vi "Metadata_Testing.vi"() -> ()   [LabVIEW 2016]
uses:
  <userlib>/LevyLab/Lockin-Multichannel/Typedefs/AO-cluster.ctl
  <userlib>/LevyLab/Lockin-Multichannel/Typedefs/AO_Amp-array.ctl
  <userlib>/LevyLab/Lockin-Multichannel/Typedefs/AO_DC-array.ctl
  <userlib>/LevyLab/Lockin-Multichannel/Typedefs/AO_f-array.ctl
  <userlib>/LevyLab/Lockin-Multichannel/Typedefs/AO_phi-array.ctl
  <userlib>/LevyLab/Lockin-Multichannel/Typedefs/Function-array.ctl
  <userlib>/LevyLab/Lockin-Multichannel/Typedefs/Function-enum.ctl
  levylab_expt_transport/src/SMOs/SweepControl/Typedefs/ScanParamters.ctl
  levylab_expt_transport/src/SMOs/SweepControl/Typedefs/Cluster - ScanParamters.ctl
  levylab_expt_transport/src/SMOs/SweepControl/Typedefs/PostAction.ctl
  levylab_expt_transport/src/SMOs/SweepControl/Typedefs/Enum - PostAction.ctl
  levylab_expt_transport/src/SMOs/SweepControl/Typedefs/ScanControl.ctl
  levylab_expt_transport/src/SMOs/SweepControl/Typedefs/Cluster - ScanControl.ctl
  levylab_expt_transport/src/SMOs/SweepControl/Typedefs/Enum - Priority.ctl
  levylab_expt_transport/src/SMOs/SweepControl/Typedefs/Enum - Action.ctl
  levylab_expt_transport/src/subVI/SweepMetadataV2.ctl
  levylab_expt_transport/src/SMOs/SweepControl/SweepControl.lvclass
panel:
  out "Sweep Metadata Cluster":T1 {"Channels: AO"."AO f (Hz)" min=0.001 max=10000.0; "Channels: AO"."AO DC (V)" format="%#_6p"; "Channels: AO"."AO amp (V)" format="%#_6p"}
  out "output cluster":T17 {"Sorted scan parameters"."?"."Rate" format="%.2f"; "Sorted scan parameters"."?"."Step" format="%#_6p"; "Sorted scan parameters"."?"."End" format="%#_6p"; "Sorted scan parameters"."?"."Start" format="%#_6p"}
  in  "<FROM SCAN CONTROL>":T18 {"Channels: AO"."AO f (Hz)" min=0.001 max=10000.0; "Channels: AO"."AO DC (V)" format="%#_6p"; "Channels: AO"."AO amp (V)" format="%#_6p"; "Scan parameters"."Rate" format="%.2f"; "Scan parameters"."Step" format="%#_6p"; "Scan parameters"."End" format="%#_6p"; "Scan parameters"."Start" format="%#_6p"}
  # "0"
  # "1"
  # "2"
  # "3"
  # "4"
  # "5"
  # "6"
  # "7"
  # "0"
  # "1"
  # "2"
  # "3"
  # "4"
  # "5"
  # "6"
  # "7"
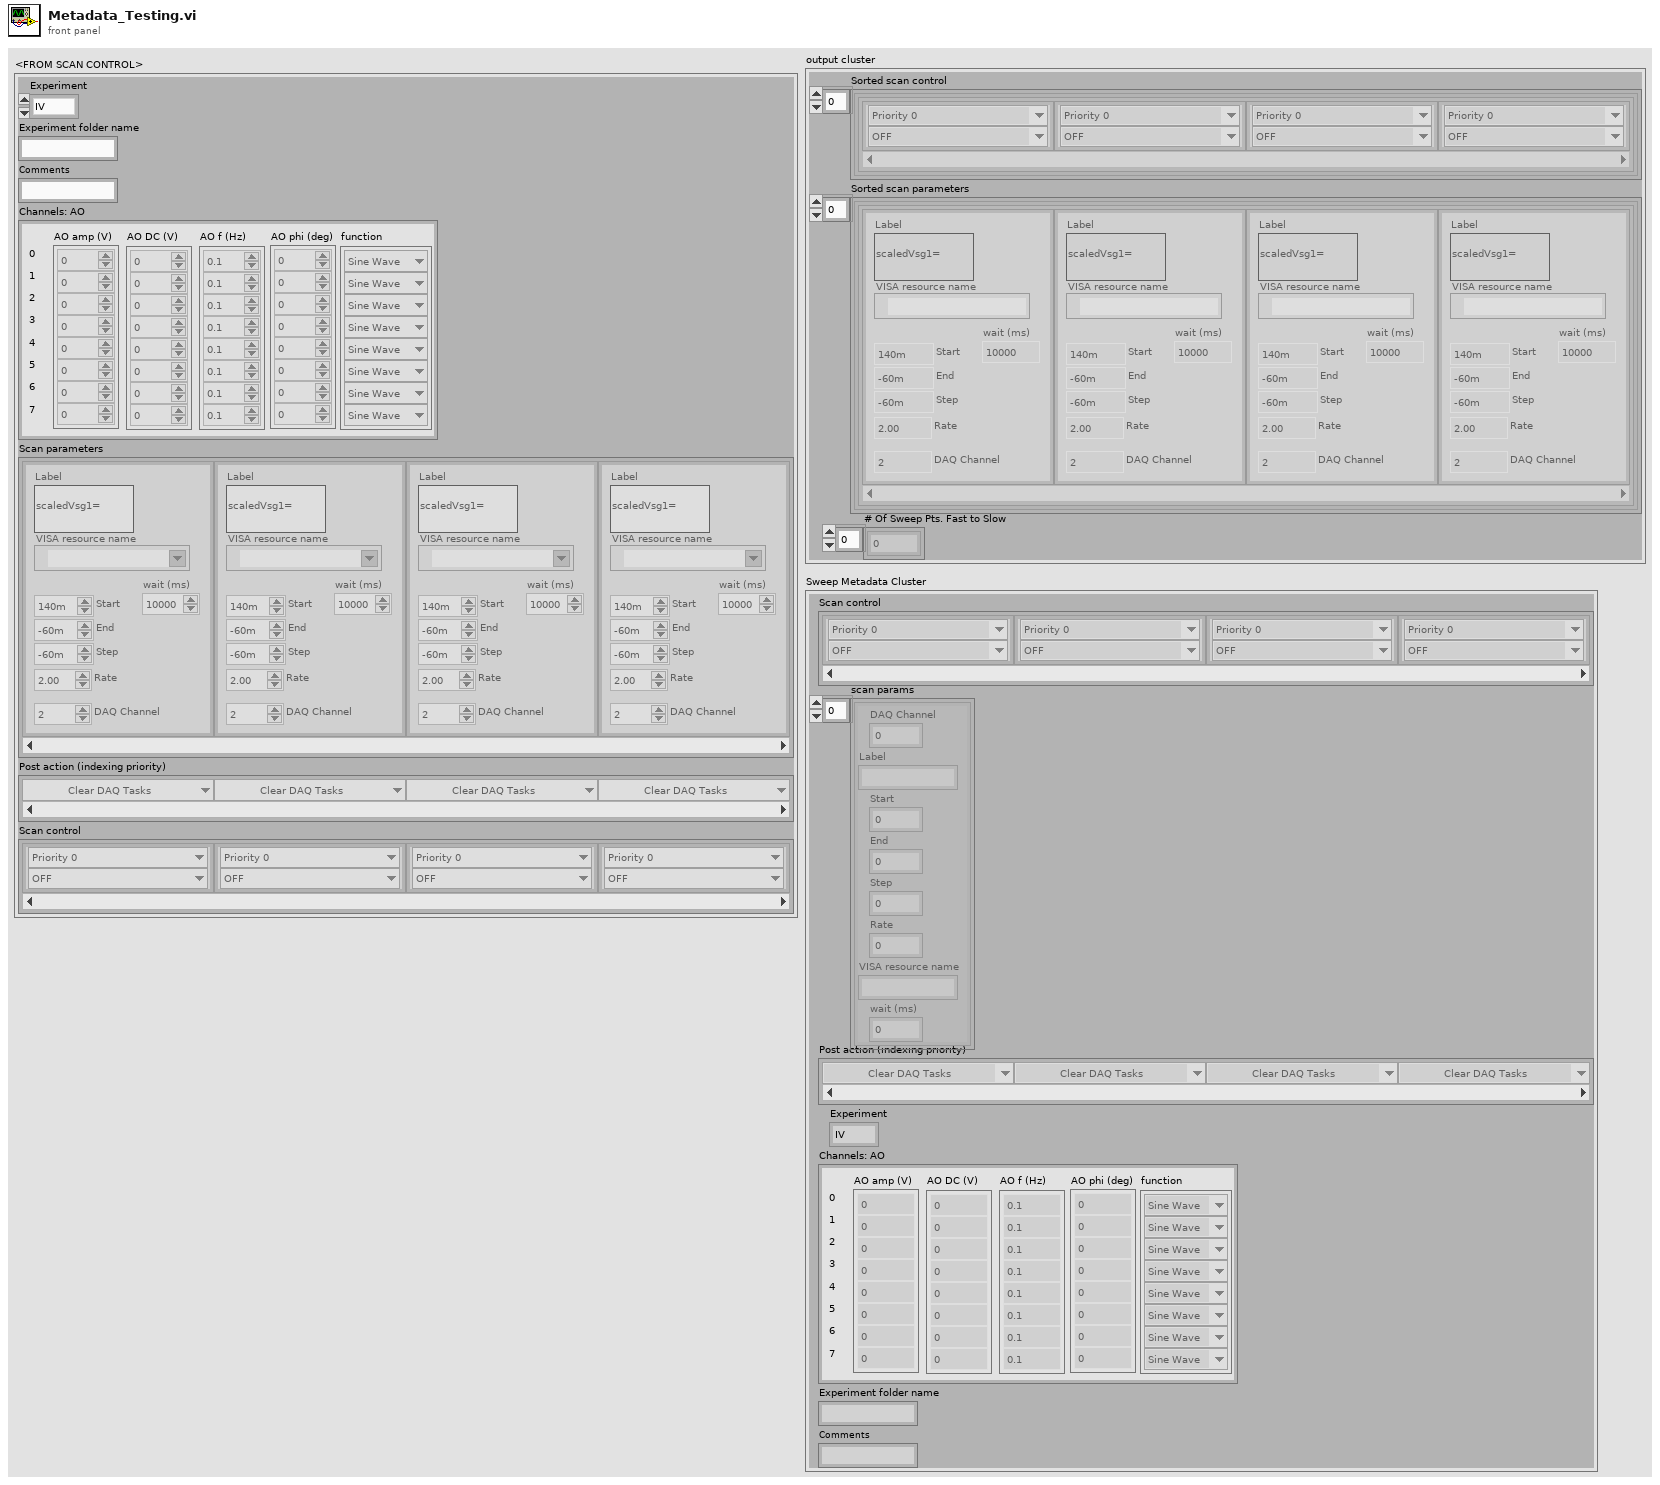
[diagram p1: front panel]
types:
  T1 = typedef "SweepMetadataV2.ctl" = cluster{"Experiment":enum16{"IV", "lockin_time", "Lockin_Vsg"}, "Experiment folder name":string, "Comments":string, "Channels: AO":T2, "Post action (indexing priority)":T9, "Scan control":T11, "scan params":cluster{"DAQ Channel":i32, "Label":string, "Start":dbl, "End":dbl, "Step":dbl, "Rate":dbl, "VISA resource name":string, "wait (ms)":u32}[]}
  T2 = typedef "AO-cluster.ctl" = cluster{"AO amp (V)":T3, "AO DC (V)":T4, "AO f (Hz)":T5, "AO phi (deg)":T6, "function":T7}
  T3 = typedef "AO_Amp-array.ctl" = dbl[]
  T4 = typedef "AO_DC-array.ctl" = dbl[]
  T5 = typedef "AO_f-array.ctl" = dbl[]
  T6 = typedef "AO_phi-array.ctl" = dbl[]
  T7 = typedef "Function-array.ctl" = T8[]
  T8 = typedef "Function-enum.ctl" = enum16{"Sine Wave", "Triangle Wave", "Square Wave", "Sawtooth Wave"}
  T9 = typedef "SweepControl.lvclass/PostAction.ctl" = T10[]
  T10 = typedef "SweepControl.lvclass/Enum - PostAction.ctl" = enum16{"Clear DAQ Tasks", "Check Temperature", "Wait", "Do Nothing"}
  T11 = typedef "SweepControl.lvclass/ScanControl.ctl" = T12[]
  T12 = typedef "SweepControl.lvclass/Cluster - ScanControl.ctl" = cluster{"Priority":T13, "Scan name":T14}
  T13 = typedef "SweepControl.lvclass/Enum - Priority.ctl" = enum16{"Priority 0", "Priority 1", "Priority 2", "Priority 3", "Priority 4", "Priority 5"}
  T14 = typedef "SweepControl.lvclass/Enum - Action.ctl" = enum16{"OFF", "DSA_Vamp", "DSA_freq", "DSA_Vsg1", "DSA_Vsg2", "DSA_Vsg3", "DAQ_Vbg", "B_Field", "Humidity", "Temp", "MW_freq1", "MW_freq2", "MW_amplitude1", "MW_amplitude2"}
  T15 = typedef "SweepControl.lvclass/ScanParamters.ctl" = T16[]
  T16 = typedef "SweepControl.lvclass/Cluster - ScanParamters.ctl" = cluster{"DAQ Channel":i32, "Label":string, "Start":dbl, "End":dbl, "Step":dbl, "Rate":dbl, "VISA resource name":refnum<visa-resource-name>, "wait (ms)":u32}
  T17 = cluster{"Sorted scan control":cluster{T11}[], "Sorted scan parameters":cluster{T15}[], "# Of Sweep Pts. Fast to Slow":i16[]}
  T18 = cluster{"Experiment":enum16{"IV", "lockin_time", "Lockin_Vsg"}, "Experiment folder name":string, "Comments":string, "Channels: AO":T2, "Scan parameters":T15, "Post action (indexing priority)":T9, "Scan control":T11}
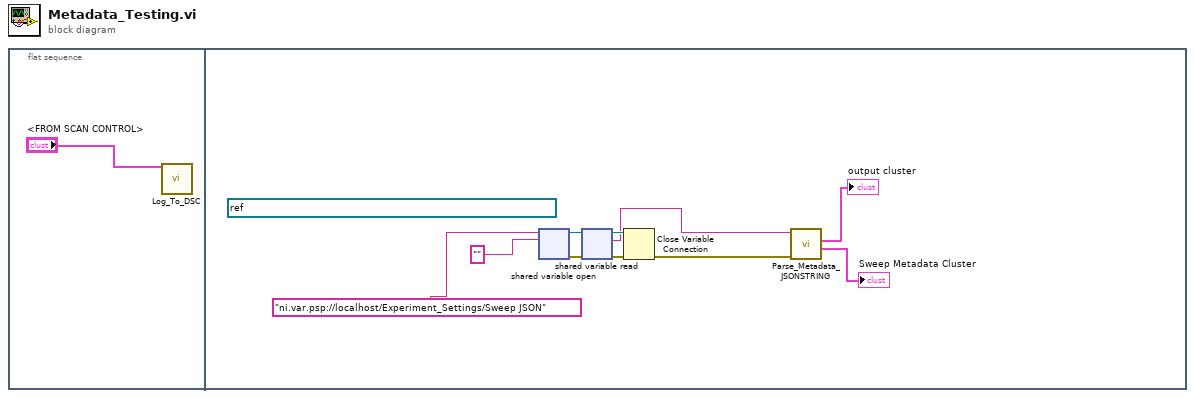
[diagram p0: block diagram]
diagram:
  n1 = flat-sequence {
    frame #0 {
      n2 = call "Log_To_DSC.vi"("Input"="<FROM SCAN CONTROL>") -> ()  [unwired: 10 in, 1 out]
    }
    frame #1 {
      (unwired) refnum<k21> "ni.var.psp://localhost/Experiment_Settings/Sweep JSON" ("shared variable refnum in")
      n3 = shared-variable-open("ni.var.psp://localhost/Experiment_Settings/Sweep JSON", "") -> (w8:refnum<k21>, w11:errorcluster)  [unwired: 2 in]
      n4 = shared-variable-read(w8, w11) -> (w9:refnum<k21>, w10:errorcluster, w6:string)  [unwired: 1 out]
      n5 = Close Variable Connection(8:w10, 11:w9) -> (0:w5:errorcluster)
      n6 = call "Parse_Metadata_JSONSTRING.vi"("error in (no error)"=w5, "JSON String"=w6) -> ("Sweep Metadata Cluster"=→"Sweep Metadata Cluster":T1, "parsed info output"=→"output cluster":T17)  [unwired: 7 in, 1 out]
    }
  }
